vi "TP1.3.vi"() -> ()   [LabVIEW 2013]
panel:
  out "Waveform Graph 2":dbl[](graph)
  in  "Frecuencia":dbl=5.0
  in  "Amplitud":dbl=10.0
  in  "Cantidad de Muestras":i32=1000
  in  "Boolean":bool
  in  "Función":bool
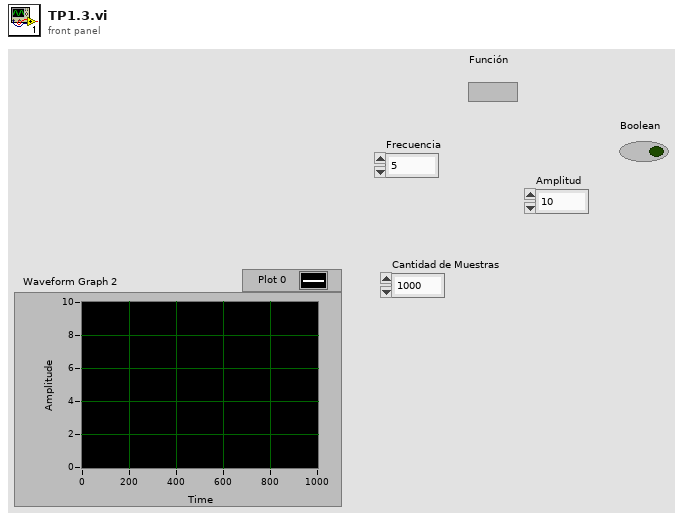
[diagram p1: front panel]
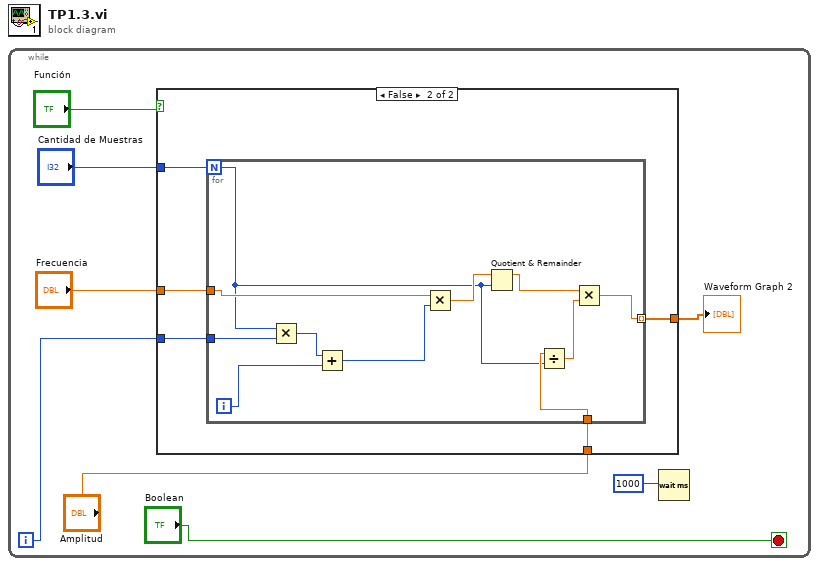
[diagram p0: block diagram]
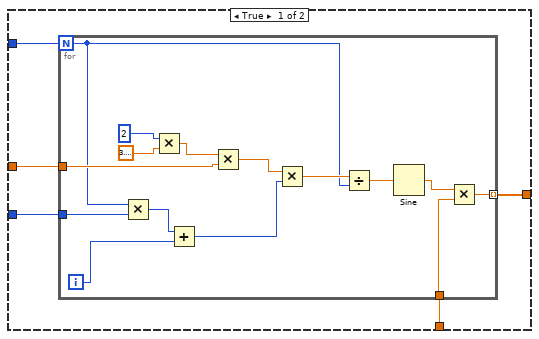
[diagram p2: hidden frame]
diagram:
  n1 = while {
    i -> [w8]
    stop <- "Boolean" stop-if-true
    n2 = case shown="False" "Función" {
      tunnel: w8 -> [w9 w31]
      tunnel: [w12 w33] -> w6
      tunnel: "Amplitud" -> [w13 w32]
      tunnel: "Cantidad de Muestras" -> [w11 w29]
      tunnel: "Frecuencia" -> [w10 w30]
      frame True {
        n3 = for {
          N: w11 -> [w17]
          tunnel: w10 -> [w22]
          tunnel: w13 -> [w21]
          tunnel: [w19] -> w12 mode=indexing
          tunnel: w9 -> [w16]
          i -> [w18]
          n4 = Multiply(x=w17, y=w16) -> (x*y=w15:i32)
          n5 = Multiply(x=2, y=3.141592653589793) -> (x*y=w26:dbl)
          n6 = Add(x=w15, y=w18) -> (x+y=w14:i32)
          n7 = Multiply(x=w26, y=w22) -> (x*y=w25:dbl)
          n8 = Multiply(x=w25, y=w14) -> (x*y=w24:dbl)
          n9 = Divide(x=w24, y=w17) -> (x/y=w23:dbl)
          n10 = Sine(x=w23) -> (sin(x)=w20:dbl)
          n11 = Multiply(x=w20, y=w21) -> (x*y=w19:dbl)
        }
      }
      frame False {
        n12 = for {
          N: w29 -> [w37]
          tunnel: w30 -> [w40]
          tunnel: w32 -> [w38]
          tunnel: [w34] -> w33 mode=indexing
          tunnel: w31 -> [w43]
          i -> [w44]
          n13 = Multiply(x=w37, y=w43) -> (x*y=w42:i32)
          n14 = Add(x=w42, y=w44) -> (x+y=w41:i32)
          n15 = Multiply(x=w40, y=w41) -> (x*y=w39:dbl)
          n16 = Quotient & Remainder(x=w39, y=w37) -> (x-y*floor(x/y)=w36:dbl)  [unwired: 1 out]
          n17 = Divide(x=w38, y=w37) -> (x/y=w35:dbl)
          n18 = Multiply(x=w36, y=w35) -> (x*y=w34:dbl)
        }
      }
    }
    "Waveform Graph 2" <- w6
    n19 = Wait (ms)(milliseconds to wait=1000) -> ()  [unwired: 1 out]
  }
